vi "Write_Data_MsgQ.vi"(8 "error in (no error)":errorcluster, 10 "Data in":string[](array[string])=[""], 11 "Command":T1) -> (0 "error out":errorcluster, 1 "timed out?":bool, 2 "ResponseAddr":string)   [LabVIEW 2019, in "MsgQ.lvlib"]
uses:
  MsgQ.lvlib
  TypeDefs/MsgQ_Commands.ctl
  TypeDefs/CommandsQ.ctl
  Service/Service.lvlib
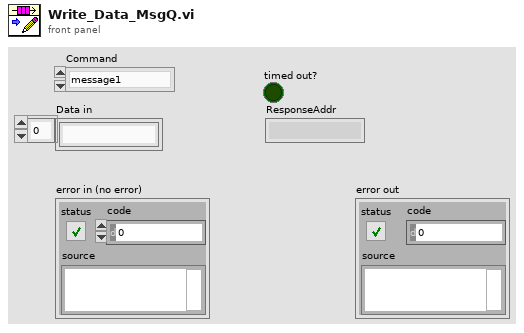
[diagram p1: front panel]
types:
  T1 = typedef "MsgQ.lvlib/MsgQ_Commands.ctl" = enum16{"message1", "message2", "message3", "generic", "transparent", "exception", "stop"}
  T2 = typedef "Service.lvlib/CommandsQ.ctl" = cluster{"cmd":T1, "data":variant, "notif":string}
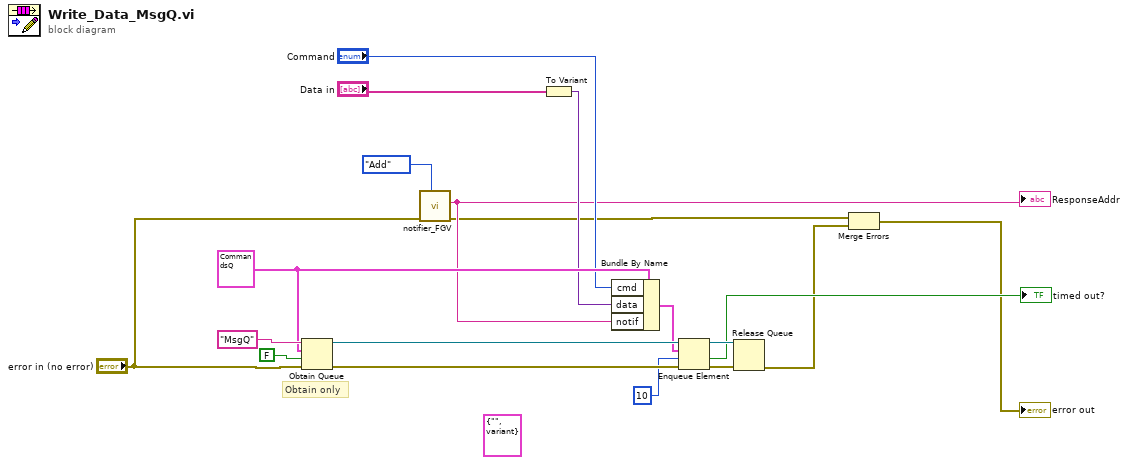
[diagram p0: block diagram]
diagram:
  w12 = T2 {"cmd"=enum."message1", "data"=variant, "notif"="notif1"}
  (unwired) cluster{enum16{""}, "element data type":variant} {enum."", "element data type"=variant}
  # "Obtain only"
  n1 = Obtain Queue(name (unnamed)="MsgQ", element data type=w12, create if not found? (T)=FALSE, error in (no error)="error in (no error)") -> (queue out=w17:refnum<queue>, error out=w15:errorcluster)  [unwired: 1 in, 1 out]
  n2 = call "notifier_FGV.vi"("Mode"=enum16{"Status", "Add", "Access", "Delete"}."Add", "error in (no error)"="error in (no error)") -> ("error out"=w1:errorcluster, "ResponseAddr out"=w2:string)  [unwired: 6 in, 2 out]
  "ResponseAddr" <- w2
  n3 = To Variant(anything="Data in") -> (Variant=w10:variant)
  n4 = Bundle By Name(cluster=w12, "cmd"="Command", "data"=w10, "notif"=w2) -> (w8:T2)
  n5 = Enqueue Element(queue=w17, element=w8, timeout in ms (-1)=10, error in (no error)=w15) -> (queue out=w16:refnum<queue>, timed out?=→"timed out?":bool, error out=w13:errorcluster)
  n6 = Release Queue(queue=w16, error in (no error)=w13) -> (error out=w6:errorcluster)  [unwired: 1 in, 2 out]
  n7 = Merge Errors(w1, w6) -> (→"error out":errorcluster)
